vi "GFITS_processOneExt_single.vi"(6 "def_timing":string="after", 9 "starting line":u16, 10 "line string":string) -> (1 "finished":bool, 2 "number of keywords":i32, 3 "Extension Keywords":string[][](table), 5 "number of before keywords":i32, 7 "Extension before keywords":string[][](array[string]))   [LabVIEW 2016]
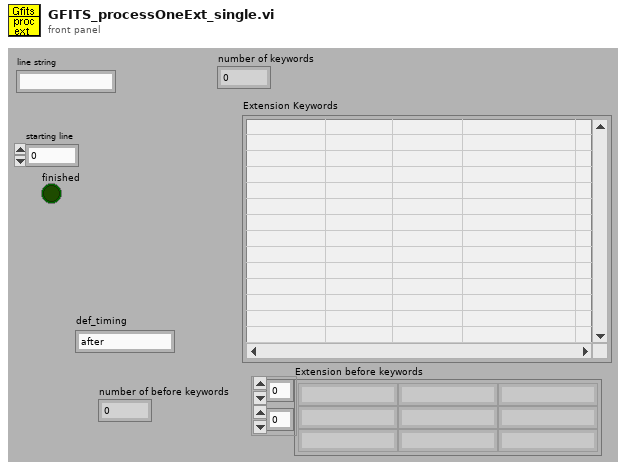
[diagram p1: front panel]
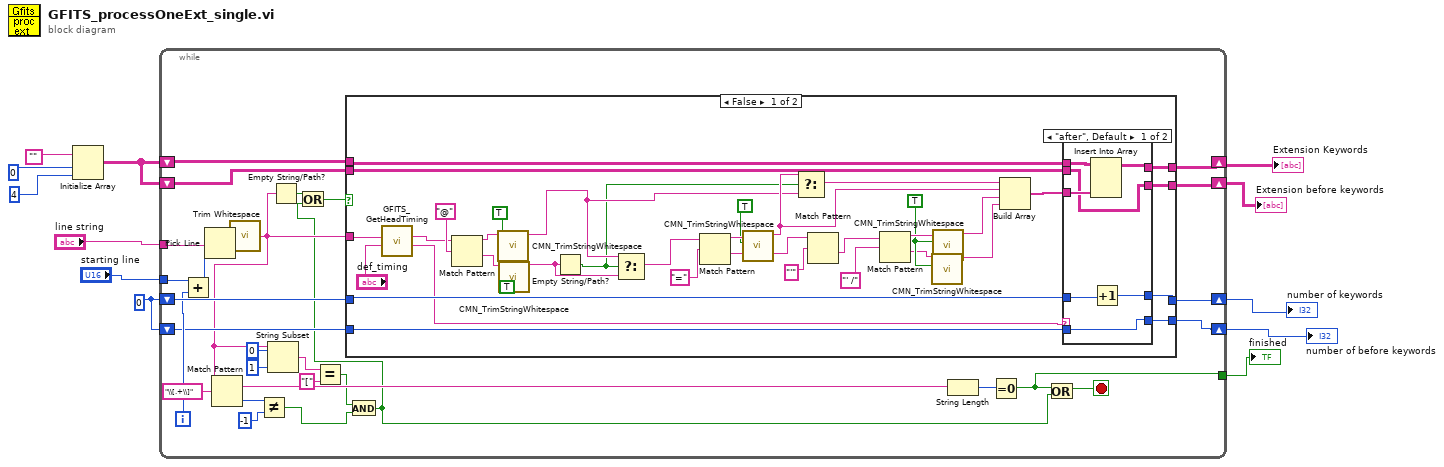
[diagram p0: block diagram]
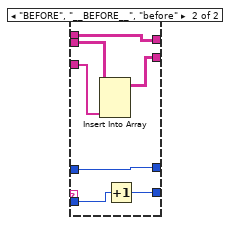
[diagram p2: hidden frame]
diagram:
  w4 = 0
  n1 = Initialize Array("", 0, 4) -> (w3:string[][])
  n2 = while {
    shift-left: w4 -> [w28]
    shift-right: [w27] -> w5
    tunnel: [w32] -> w10
    tunnel: "starting line" -> [w37]
    shift-left: w3 -> [w39]
    shift-right: [w38] -> w6
    tunnel: "line string" -> [w41]
    shift-right: [w24] -> w1
    shift-left: w4 -> [w25]
    shift-right: [w23] -> w2
    shift-left: w3 -> [w22]
    i -> [w26]
    stop <- w35 stop-if-true
    n3 = Add(x=w37, y=w26) -> (x+y=w36:i32)
    n4 = Pick Line(multi-line string=w41, line index=w36) -> (output string=w30:string)  [unwired: 1 out]
    n5 = call <vilib>:"Trim Whitespace.vi"("string"=w30) -> ("trimmed string"=w20:string)  [unwired: 1 in]
    n6 = Match Pattern(string=w20, regular expression="\\[.+\\]") -> (offset past match=w34:i32)  [unwired: 4 out]
    n7 = Not Equal?(x=w34, y=-1) -> (x != y?=w15:bool)
    n8 = String Subset(string=w20, offset (0)=0, length (rest)=1 ("length (rest)")) -> (substring=w18:string)
    n9 = Empty String/Path?(string/path=w20) -> (empty?=w31:bool)
    n10 = Equal?(x=w18, y="[") -> (x = y?=w16:bool)
    n11 = And(x=w16, y=w15) -> (x .and. y?=w13:bool)
    n12 = Or(x=w31, y=w13) -> (x .or. y?=w29:bool)
    n13 = case shown="False" w29 {
      tunnel: w39 -> [w64 w95]
      tunnel: [w63 w95] -> w38
      tunnel: w28 -> [w51 w94]
      tunnel: [w50 w94] -> w27
      tunnel: w20 -> [w49 _]
      tunnel: w25 -> [w45 w92]
      tunnel: [w44 w92] -> w24
      tunnel: [w43 w93] -> w23
      tunnel: w22 -> [w42 w93]
      frame False {
        w69 = TRUE ("Both Ends?(F)")
        n14 = call "GFITS_GetHeadTiming.vi"("def_timing"="def_timing", "line In"=w49) -> ("head_tim"=w46:string, "line out"=w48:string)  [unwired: 8 out]
        n15 = Match Pattern(string=w48, regular expression="@") -> (before substring=w58:string, after substring=w60:string)  [unwired: 3 out]
        n16 = call "CMN_TrimStringWhitespace.vi"("Both Ends?(T)"=TRUE ("Both Ends?(F)"), "string"=w58) -> ("trimmed string"=w54:string)  [unwired: 8 out]
        n17 = call "CMN_TrimStringWhitespace.vi"("Both Ends?(T)"=TRUE ("Both Ends?(F)"), "string"=w60) -> ("trimmed string"=w57:string)  [unwired: 8 out]
        n18 = Empty String/Path?(string/path=w57) -> (empty?=w52:bool)
        n19 = Select(t=w54, s=w52, f=w57) -> (s? t:f=w56:string)
        n20 = Match Pattern(string=w56, regular expression="=") -> (before substring=w76:string, after substring=w75:string)  [unwired: 3 out]
        n21 = call "CMN_TrimStringWhitespace.vi"("Both Ends?(T)"=TRUE ("Both Ends?(F)"), "string"=w76) -> ("trimmed string"=w55:string)  [unwired: 8 out]
        n22 = Select(t=w55, s=w52, f=w54) -> (s? t:f=w53:string)
        n23 = Match Pattern(string=w75, regular expression="'") -> (after substring=w73:string)  [unwired: 4 out]
        n24 = Match Pattern(string=w73, regular expression="' /") -> (before substring=w71:string, after substring=w68:string)  [unwired: 3 out]
        n25 = call "CMN_TrimStringWhitespace.vi"("Both Ends?(T)"=w69, "string"=w68) -> ("trimmed string"=w66:string)  [unwired: 8 out]
        n26 = call "CMN_TrimStringWhitespace.vi"("Both Ends?(T)"=w69, "string"=w71) -> ("trimmed string"=w67:string)  [unwired: 8 out]
        n27 = Build Array(w53, w55, w67, w66) -> (w65:string[])
        n28 = case shown="\"after\", Default" w46 {
          tunnel: w65 -> [w84 w87]
          tunnel: w64 -> [w83 w91]
          tunnel: [w82 w91] -> w63
          tunnel: w51 -> [w81 w90]
          tunnel: [w80 w90] -> w50
          tunnel: w45 -> [w78 w89]
          tunnel: [w78 w88] -> w44
          tunnel: [w79 w86] -> w43
          tunnel: w42 -> [w79 w85]
          frame "after", Default {
            n29 = Insert Into Array(array=w83, new element=w84) -> (w82:string[][])  [unwired: 2 in]
            n30 = Increment(x=w81) -> (x+1=w80:i32)
          }
          frame "BEFORE", "__BEFORE__", "before" {
            n31 = Insert Into Array(array=w85, new element=w87) -> (w86:string[][])  [unwired: 2 in]
            n32 = Increment(x=w89) -> (x+1=w88:i32)
          }
        }
      }
      frame True {
      }
    }
    n33 = String Length(string=w20) -> (length=w40:i32)
    n34 = Equal To 0?(x=w40) -> (x = 0?=w32:bool)
    n35 = Or(x=w32, y=w13) -> (x .or. y?=w35:bool)
  }
  "number of keywords" <- w5
  "finished" <- w10
  "Extension Keywords" <- w6
  "Extension before keywords" <- w2
  "number of before keywords" <- w1
